vi "Start or Stop Cryo.vi"(8 "error in":errorcluster, 10 "VISA resource name":refnum<visa-resource-name>, 11 "State":enum16{"Start", "Stop"}(ring)) -> (0 "error out":errorcluster, 3 "VISA resource name out":refnum<visa-resource-name>)   [LabVIEW 2021]
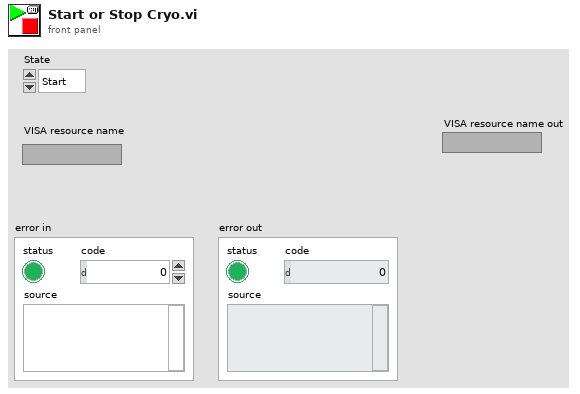
[diagram p1: front panel]
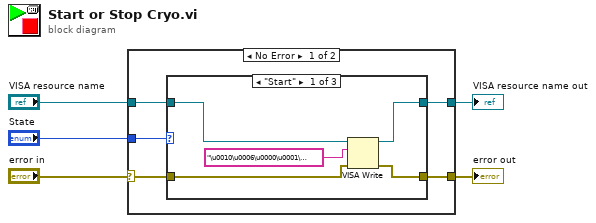
[diagram p0: block diagram]
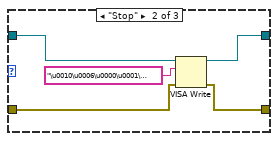
[diagram p2: hidden frame]
diagram:
  n1 = case shown="No Error" "error in" {
    selector: "error in" -> [w6 w24]
    tunnel: [w7 w24] -> w4
    tunnel: "State" -> [w10 _]
    tunnel: "VISA resource name" -> [w9 w23]
    tunnel: [w8 w23] -> w1
    frame No Error {
      n2 = case shown="\"Start\"" w10 {
        tunnel: w9 -> [w15 w20 w22]
        tunnel: [w11 w16 w22] -> w8
        tunnel: [w13 w17 w21] -> w7
        tunnel: w6 -> [w14 w19 w21]
        frame "Start" {
          n3 = VISA Write(VISA resource name=w15, write buffer="\u0010\u0006\u0000\u0001\u0000\u0001\u001a‹", error in (no error)=w14) -> (VISA resource name out=w11:refnum<visa-resource-name>, error out=w13:errorcluster)  [unwired: 1 out]
        }
        frame "Stop" {
          n4 = VISA Write(VISA resource name=w20, write buffer="\u0010\u0006\u0000\u0001\u0000ÿ›\u000b", error in (no error)=w19) -> (VISA resource name out=w16:refnum<visa-resource-name>, error out=w17:errorcluster)  [unwired: 1 out]
        }
        frame Default {
        }
      }
    }
    frame Error {
    }
  }
  "error out" <- w4
  "VISA resource name out" <- w1
